vi "Any two true.vi"(10 "Array in":bool[](array[boolean])) -> (2 "Any two true?":bool)   [LabVIEW 2012]
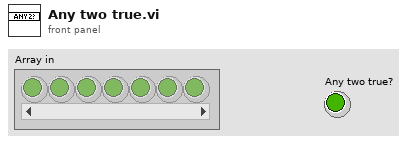
[diagram p1: front panel]
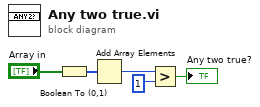
[diagram p0: block diagram]
diagram:
  n1 = Boolean To (0,1)(Boolean="Array in") -> (0, 1=w4:i16[])
  n2 = Add Array Elements(numeric array=w4) -> (sum=w3:i16)
  n3 = Greater?(x=w3, y=i16 1) -> (0:→"Any two true?":bool)
